vi "Record Fluidics Data.vi"() -> ()   [LabVIEW 2016]
uses:
  <vilib>/Platform/TimedLoop/XDataNode/timing_clust.ctl
  <vilib>/Platform/TimedLoop/XDataNode/nitl_modes.ctl
  <vilib>/Platform/TimedLoop/XDataNode/wakeup.ctl
  <vilib>/Utility/file.llb/Write Delimited Spreadsheet (string).vi
  <vilib>/Utility/file.llb/Write Delimited Spreadsheet (DBL).vi
  <vilib>/platform/TimedLoop/XDataNode/XDataNode.xnode
  <vilib>/Platform/TimedLoop/XDataNode/XDNodeRunTimeDep.lvlib
panel:
  in  "US Cmd":i32
  in  "Vacuum Cmd":sgl
  in  "Irrigation Height":i32
  out "Elaspsed Time":sgl
  in  "File Path":path=path "C:/FluidicsData1.txt"
  out "File Exists":bool
  in  "Seconds of Data":sgl=10.0
  in  "Take IOP Data":bool
  in  "Program Stop":bool
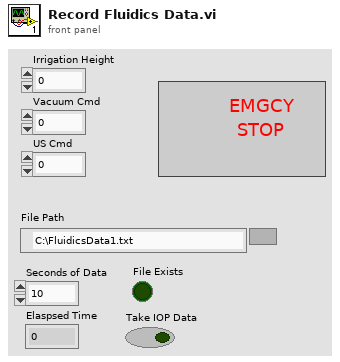
[diagram p1: front panel]
types:
  T1 = typedef "XDNodeRunTimeDep.lvlib/timing_clust.ctl" = cluster{"Expected End [f-1]":u64, "Actual End [f-1]":u64, "Finished Late? [f-1]":bool, "Expected End [i-1]":u64, "Actual End [i-1]":u64, "Finished Late? [i-1]":bool, "Expected Start [i]":u64, "Actual Start [i]":u64, "Expected Start [f]":u64, "Actual Start [f]":u64, "Source Name":string, "Structure Name":string, "Period":i64, "Deadline":i64, "Offset":i64, "Start":i64, "Priority":i32, "Timeout":i32, "Mode":T2, "Wakeup Reason":T3, "Error":errorcluster, "Source Type":string, "Secondary Source Type":string, "Global End Time":u64, "Global Start Time":u64, "Frame Duration":u64, "Iteration Duration":u64, "Assigned CPU":i32, "I/O Scan Engine Mode":u32}
  T2 = typedef "XDNodeRunTimeDep.lvlib/nitl_modes.ctl" = enum32{"No Change", "Process missed periods, maintain original phase", "Discard missed periods, maintain original phase", "Process missed periods, ignore original phase", "Discard missed periods, ignore original phase"}
  T3 = typedef "XDNodeRunTimeDep.lvlib/wakeup.ctl" = enum32{"Normal", "Aborted", "Asynchronous wakeup", "Timing source error", "Timed loop error", "Timeout"}
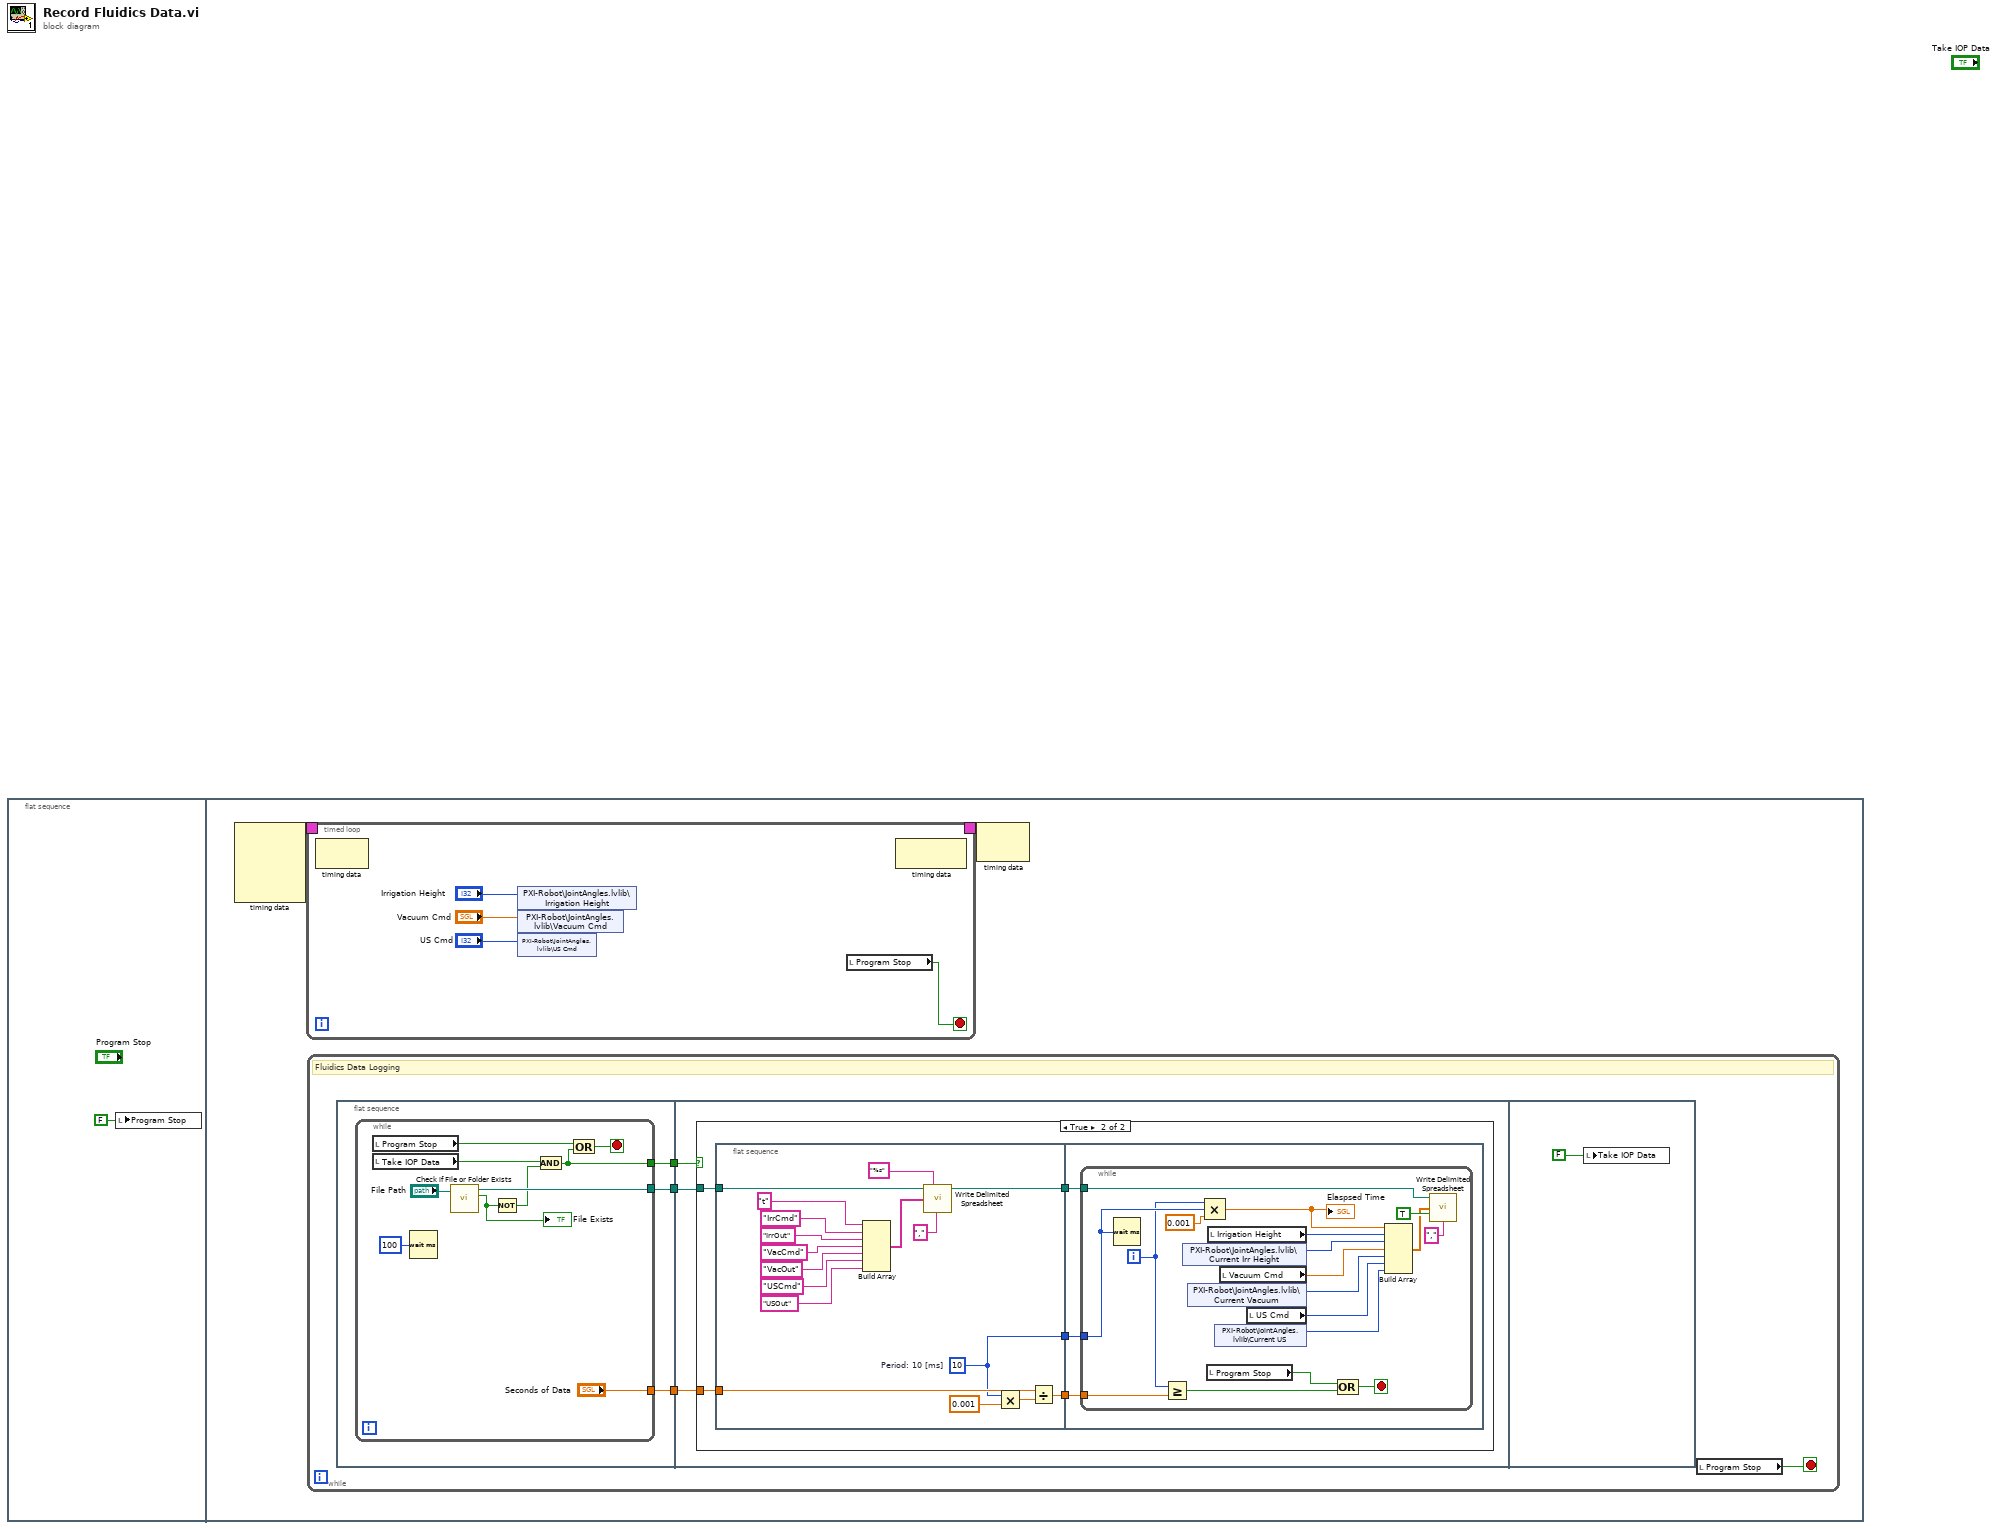
[diagram p0: block diagram]
diagram:
  n1 = flat-sequence {
    frame #0 {
      n2 = local write "Program Stop"(FALSE ("Program Stop")) -> ()
    }
    frame #1 {
      n3 = node-c288() -> (w3:T1)  [unwired: 4 in]
      n4 = timed-loop {
        timing: w3 -> [_]
        timing-out: [_] -> w2
        stop <- w4 stop-if-true
        n5 = node-c288() -> ()  [unwired: 1 in, 1 out]
        n6 = shared-variable "PXI-Robot\\JointAngles.lvlib\\Irrigation Height"("Irrigation Height") -> ()  [unwired: 1 in, 1 out]
        n7 = shared-variable "PXI-Robot\\JointAngles.lvlib\\Vacuum Cmd"("Vacuum Cmd") -> ()  [unwired: 1 in, 1 out]
        n8 = shared-variable "PXI-Robot\\JointAngles.lvlib\\US Cmd"("US Cmd") -> ()  [unwired: 1 in, 1 out]
        n9 = local read "Program Stop"() -> (w4:bool)
        n10 = node-c288() -> ()  [unwired: 1 in, 1 out]
      }
      n11 = while {
        stop <- w12 stop-if-true
        # "Fluidics Data Logging"
        n12 = flat-sequence {
          tunnel: [w16] -> w15
          tunnel: [w18] -> w14
          tunnel: [w17] -> w13
          tunnel: w15 -> [w31]
          tunnel: w14 -> [w30]
          tunnel: w13 -> [w29]
          frame #0 {
            n13 = while {
              tunnel: [w27] -> w18
              tunnel: ["Seconds of Data"] -> w17
              tunnel: [w25] -> w16
              stop <- w28 stop-if-true
              n14 = local read "Program Stop"() -> (w21:bool)
              n15 = local read "Take IOP Data"() -> (w24:bool)
              n16 = Wait (ms)(milliseconds to wait=u32 100) -> ()  [unwired: 1 out]
              n17 = call <vilib>:"Check if File or Folder Exists.vi"("path"="File Path") -> ("file or folder exists?"=w20:bool, "dup path"=w27:path)  [unwired: 8 in, 1 out]
              "File Exists" <- w20
              n18 = Not(x=w20) -> (.not. x?=w26:bool)
              n19 = And(x=w24, y=w26) -> (x .and. y?=w25:bool)
              n20 = Compound Arithmetic op=OR(w21, w25) -> (w28:bool)
            }
          }
          frame #1 {
            n21 = case shown="True" w31 {
              tunnel: w30 -> [_ w36]
              tunnel: w29 -> [_ w33]
              frame False {
              }
              frame True {
                n22 = flat-sequence {
                  tunnel: w36 -> [w43]
                  tunnel: [w41] -> w35
                  tunnel: [w37] -> w34
                  tunnel: w33 -> [w51]
                  tunnel: [w49] -> w32
                  tunnel: w35 -> [w56]
                  tunnel: w34 -> [w55]
                  tunnel: w32 -> [w54]
                  frame #0 {
                    w37 = 10  # Period: 10 [ms]
                    n23 = Build Array("t" ("delimiter (\\t)"), "IrrCmd" ("delimiter (\\t)"), "IrrOut" ("delimiter (\\t)"), "VacCmd" ("delimiter (\\t)"), "VacOut" ("delimiter (\\t)"), "USCmd" ("delimiter (\\t)"), "USOut" ("delimiter (\\t)")) -> (w40:string[])
                    n24 = call-poly <vilib>:"Write Delimited Spreadsheet.vi"("file path (dialog if empty)"=w43, "format (%s)"="%s", "1D data"=w40, "delimiter (\\t)"="," ("delimiter (\\t)")) -> ("new file path (Not A Path if cancelled)"=w41:path)  [unwired: 10 in, 1 out]
                    n25 = Multiply(x=w37, y=0.001) -> (x*y=w50:dbl)
                    n26 = Divide(x=w51, y=w50) -> (x/y=w49:dbl)
                  }
                  frame #1 {
                    n27 = while {
                      tunnel: w56 -> [w68]
                      tunnel: w55 -> [w72]
                      tunnel: w54 -> [w70]
                      i -> [w71]
                      stop <- w74 stop-if-true
                      n28 = Wait (ms)(milliseconds to wait=w72) -> ()  [unwired: 1 out]
                      n29 = Greater Or Equal?(x=w71, y=w70) -> (x >= y?=w69:bool)
                      n30 = shared-variable "PXI-Robot\\JointAngles.lvlib\\Current Irr Height"() -> (w59:i32)  [unwired: 1 in, 1 out]
                      n31 = shared-variable "PXI-Robot\\JointAngles.lvlib\\Current Vacuum"() -> (w58:i32)  [unwired: 1 in, 1 out]
                      n32 = Compound Arithmetic op=MULTIPLY(w71, w72, 0.001 ("y")) -> (w62:dbl)
                      "Elaspsed Time" <- w62
                      n33 = local read "Program Stop"() -> (w63:bool)
                      n34 = local read "Irrigation Height"() -> (w60:i32)
                      n35 = shared-variable "PXI-Robot\\JointAngles.lvlib\\Current US"() -> (w57:i32)  [unwired: 1 in, 1 out]
                      n36 = local read "Vacuum Cmd"() -> (w64:sgl)
                      n37 = local read "US Cmd"() -> (w61:i32)
                      n38 = Compound Arithmetic op=OR(w63, w69) -> (w74:bool)
                      n39 = Build Array(w62, w60, w59, w64, w58, w61, w57) -> (w66:dbl[])
                      n40 = call-poly <vilib>:"Write Delimited Spreadsheet.vi"("file path (dialog if empty)"=w68, "1D data"=w66, "append to file? (new file:F)"=TRUE, "delimiter (\\t)"="," ("delimiter (\\t)")) -> ()  [unwired: 10 in, 2 out]
                    }
                  }
                }
              }
            }
          }
          frame #2 {
            n41 = local write "Take IOP Data"(FALSE) -> ()
          }
        }
        n42 = local read "Program Stop"() -> (w12:bool)
      }
      n43 = node-c288(w2) -> ()  [unwired: 1 out]
    }
  }
